vi "SR430_id_query.vi"(0 "address":T1, 5 "error in (no error)":errorcluster) -> (14 "address out":T1, 16 "identification string":string, 19 "error out":errorcluster)   [LabVIEW 2015, in "SR430Driver.lvlib"]
doc: "Queries the unit for its ID.\n\nCopyright (C)\nGesellschaft für Schwerionenforschung, GSI\nPlanckstr. 1\n64291 Darmstadt\nGermany\n\nContact: D.Beck@gsi.de \n\nThis program is free software; you can redistribute it and/or modify it under the terms of the \nGNU General Public License as published by the Free Software Foundation; either version 2 of the license, or (at your option) any later version.\n\nThis program is distributed in the hope that it will be useful, but WITHOUT ANY WARRANTY; without even the implied warranty of MERCHANTABILITY or FITNESS FOR A PARTICULAR PURPOSE. See the GNU General License for more details (http://www.gnu.org).\n\nGesellschaft für Schwerionenforschung, GSI\nPlanckstr. 1, 64291 Darmstadt, Germany\nFor all questions and ideas contact: M.Richter@gsi.de, K.Poppensieker, H.Brand@gsi.de or D.Beck@gsi.de.\nLast update: 11-APR-2002"
uses:
  SR430Driver.lvlib
  SR430_VISA Control.ctl
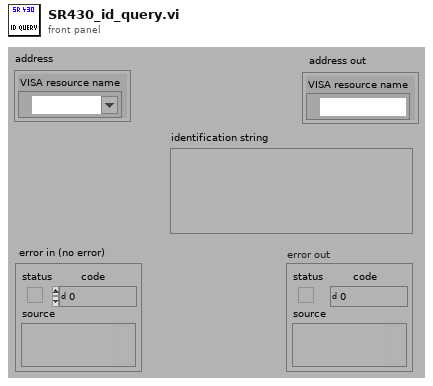
[diagram p1: front panel]
types:
  T1 = typedef "SR430Driver.lvlib/SR430_VISA Control.ctl" = cluster{"VISA resource name":refnum<visa-resource-name>}
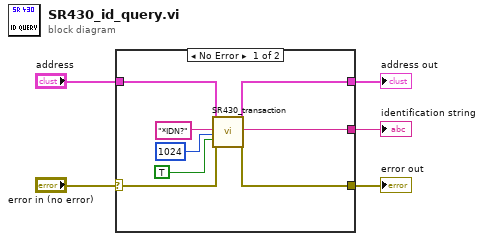
[diagram p0: block diagram]
diagram:
  n1 = case shown="No Error" "error in (no error)" {
    selector: "error in (no error)" -> [w13 w15]
    tunnel: [w12 w15] -> w2
    tunnel: "address" -> [w11 w14]
    tunnel: [w10 w14] -> w3
    tunnel: [w6 _] -> w1
    frame No Error {
      n2 = call "SR430_transaction.vi"("SR430 VISA Cluster"=w11, "SR430 Command String"="*IDN?" ("write buffer"), "Bytes to read (1024)"=u32 1024, "Read (FALSE)"=TRUE ("Read"), "error in (no error)"=w13) -> ("dup SR430 VISA Cluster"=w10:T1, "SR430 Response"=w6:string, "error out"=w12:errorcluster)  [unwired: 11 in, 1 out]
    }
    frame Error {
    }
  }
  "address out" <- w3
  "error out" <- w2
  "identification string" <- w1
